vi "System Message Destinations (SubVI).vi"(7 "Queue in":refnum<queue>, 8 "error in (no error)":errorcluster) -> ()   [LabVIEW 2019]
doc: "Takes the Messenger Queue Wire as input. Queue Wire must contain the properly formated system message cluster. \n\nThis VI runs continuously during MODAQ execution and actions messages placed in the queue by various processes within MODAQ. Based on the message contents, this VI can write entries to the system log, send an email alert, or both. Default behavior is to log all messages. In some instances it may be better to manage the snoozes at the point of message orign, since this would reduce message queue traffic and FPGA calls for the timestamp. \n\nTo avoid excessive, repetitive entries in the system log and email messages, users can enable a snooze function. Users can specify number of seconds to snooze messages, but default is 60 seconds if left unset. The snoozer sets separate timers for each caller based on the Message Tag attribute. \n\n2020 NREL"
uses:
  Globals and Definitions/System Message.ctl
  Globals and Definitions/RT Globals RD v1.0.vi
  Globals and Definitions/Initialization Globals.vi
panel:
  out "error out":errorcluster
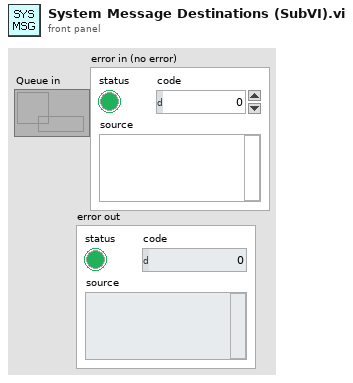
[diagram p1: front panel]
types:
  T1 = typedef "System Message.ctl" = cluster{"Message Tag":string, "Message Body":string, "Snooze Time (s)":dbl, "Snooze Alert?":bool, "Log Event?":bool, "Send Email":i32}
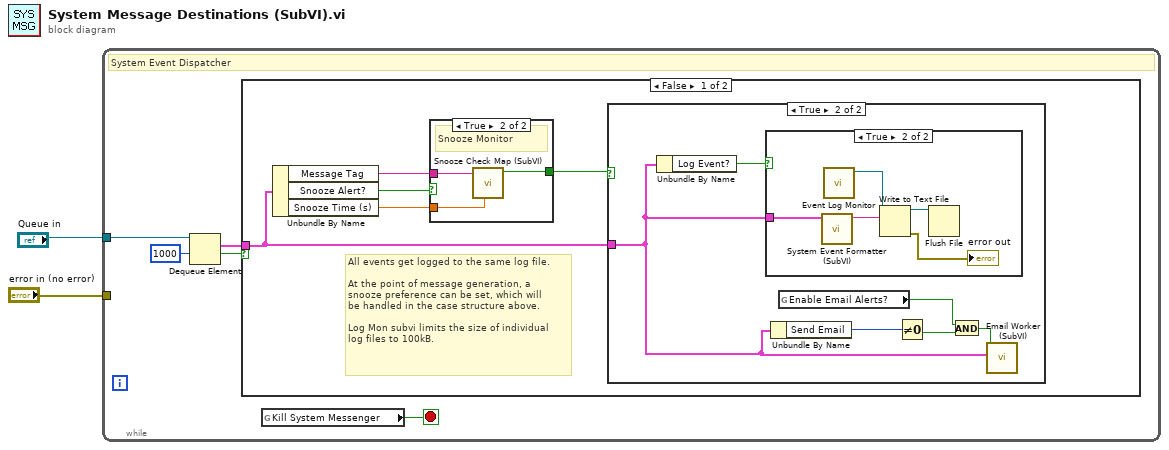
[diagram p0: block diagram]
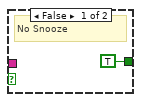
[diagram p2: hidden frame]
diagram:
  n1 = while {
    tunnel: "Queue in" -> [w7]
    tunnel: "error in (no error)" -> [_]
    stop <- w5 stop-if-true
    # "System Event Dispatcher"
    n2 = Dequeue Element(queue=w7, timeout in ms (-1)=1000) -> (element=w6:T1, timed out?=w4:bool)  [unwired: 1 in, 2 out]
    n3 = case shown="False" w4 {
      tunnel: w6 -> [w12 _]
      frame False {
        # "All events get logged to the same log file. \n\nAt the point of message generation, a \nsnooze preference can be set, which will\nbe handled in the case structure above.\n\nLog Mon subvi limits the size of individual\nlog files to 100kB."
        n4 = Unbundle By Name(w12) -> ("Message Tag"=w10:string, "Snooze Alert?"=w11:bool, "Snooze Time (s)"=w9:dbl)
        n5 = case shown="True" w11 {
          tunnel: w10 -> [_ w15]
          tunnel: w9 -> [_ w16]
          tunnel: [TRUE ("Snooze Expired?") w14] -> w8
          frame False {
            # "No Snooze"
          }
          frame True {
            # "Snooze Monitor"
            n6 = call "Snooze Check Map (SubVI).vi"("Snooze Time (s)"=w16, "key"=w15) -> ("Snooze Expired?"=w14:bool)  [unwired: 9 in]
          }
        }
        n7 = case shown="True" w8 {
          tunnel: w12 -> [_ w17]
          frame False {
          }
          frame True {
            n8 = Unbundle By Name(w17) -> ("Log Event?"=w22:bool)
            n9 = case shown="True" w22 {
              tunnel: w17 -> [_ w26]
              frame False {
              }
              frame True {
                n10 = call "System Event Formatter (SubVI).vi"("Message Cluster In"=w26) -> ("Log Message"=w25:string)  [unwired: 10 in]
                n11 = call "Event Log Monitor.vi"() -> ("Log File Refnum"=w24:refnum<file>)  [unwired: 10 in, 1 out]
                n12 = Write to Text File(file (use dialog)=w24, text=w25) -> (refnum out=w27:refnum<file>, error out=→"error out":errorcluster)  [unwired: 2 in, 1 out]
                n13 = Flush File(refnum=w27) -> ()  [unwired: 1 in, 2 out]
              }
            }
            n14 = Unbundle By Name(w17) -> ("Send Email"=w21:i32)
            n15 = global read "Initialization Globals.vi" "Enable Email Alerts?"() -> (w20:bool)
            n16 = Not Equal To 0?(x=w21) -> (x != 0?=w19:bool)
            n17 = And(x=w20, y=w19) -> (x .and. y?=w18:bool)
            n18 = call "Email Worker (SubVI).vi"("Message Cluster"=w17, "Send Email?"=w18) -> ()  [unwired: 10 in]
          }
        }
      }
      frame True {
      }
    }
    n19 = global read "RT Globals RD v1.0.vi" "Kill System Messenger"() -> (w5:bool)
  }
